vi "Test PieChart and Legend.vi"() -> ()   [LabVIEW 2020]
uses:
  Piechart Class/Pie Slice.ctl
  <vilib>/Utility/miscctls.llb/LVRowAndColumnTypeDef.ctl
  Piechart Class/PieChart.lvclass
panel:
  in  "Show/Hide Title":bool
  in  "Show/Hide Legend":bool
  in  "Selection":i32 min=-1 max=9
  out "Pie Chart":picture
  in  "Multicolumn Listbox":i32(listbox)
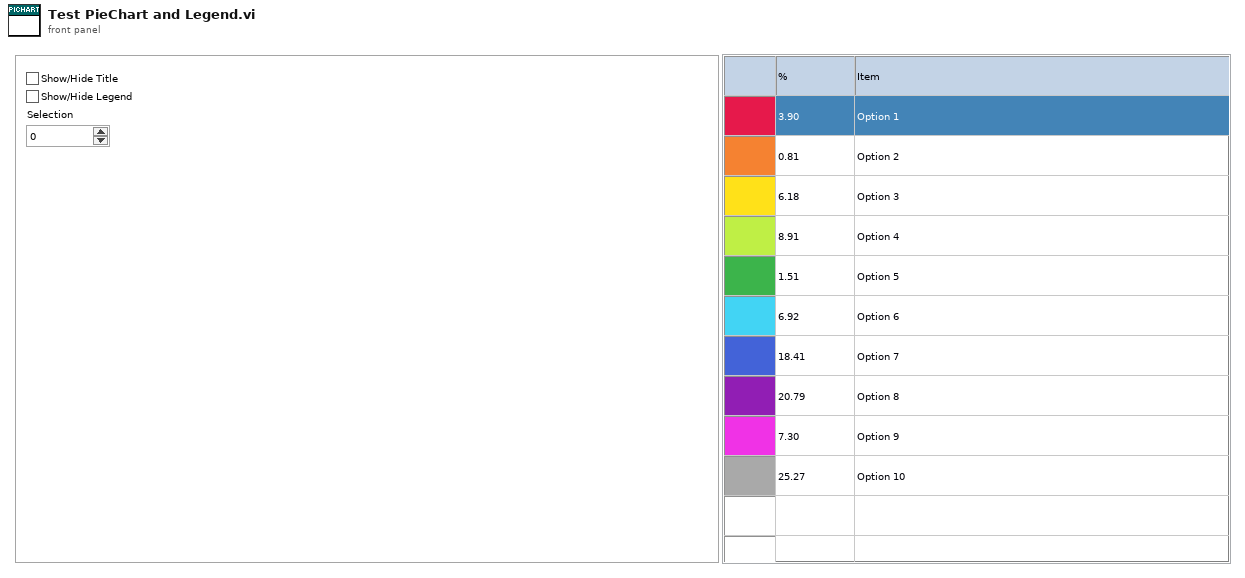
[diagram p1: front panel]
types:
  T1 = typedef "LVRowAndColumnTypeDef.ctl" = cluster{"Row":i32, "Column":i32}
  T2 = typedef "PieChart.lvclass/Pie Slice.ctl" = cluster{"Value":dbl, "Label":string}
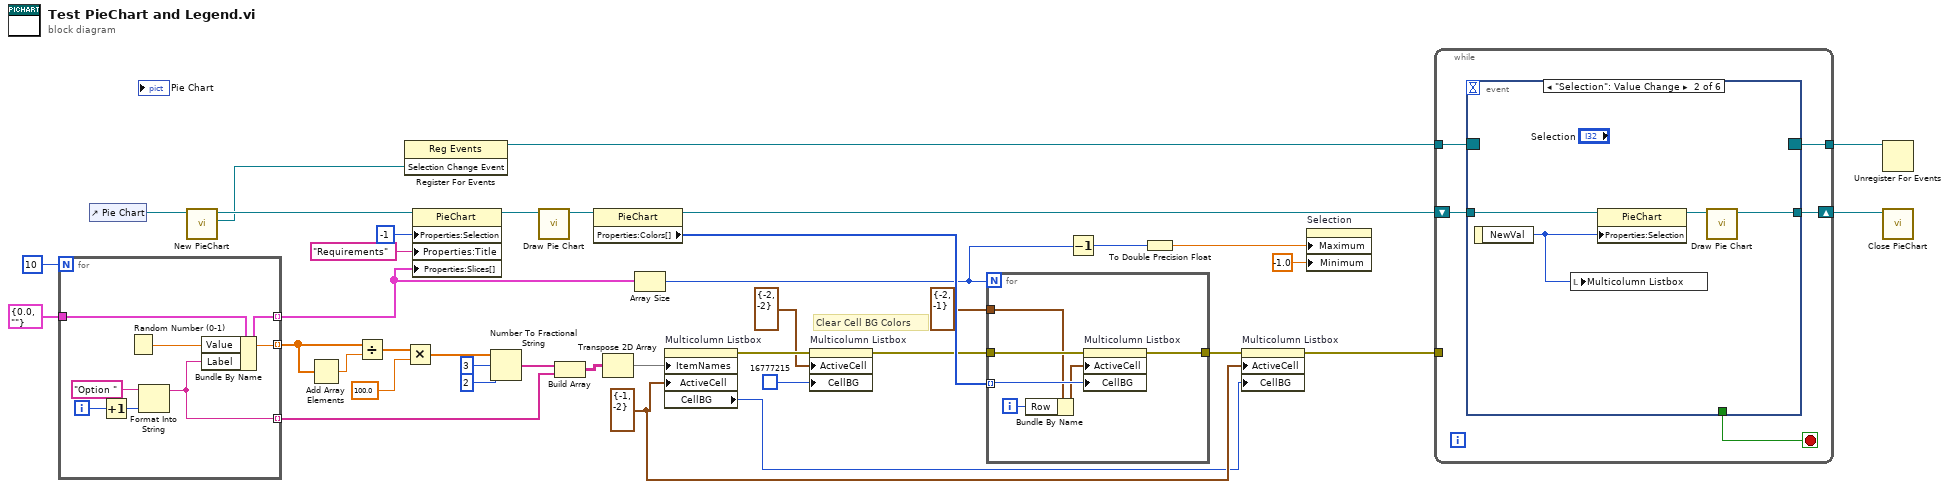
[diagram p0: block diagram]
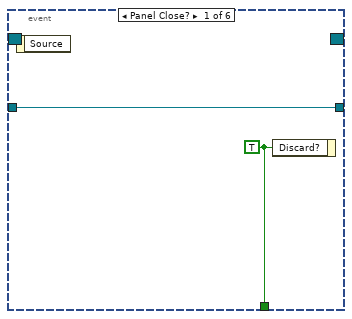
[diagram p2: hidden frame]
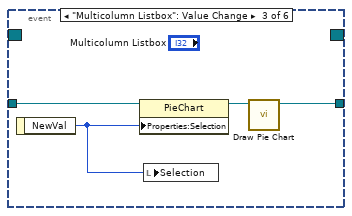
[diagram p3: hidden frame]
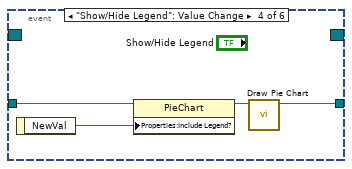
[diagram p4: hidden frame]
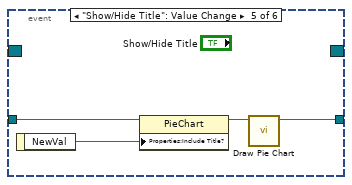
[diagram p5: hidden frame]
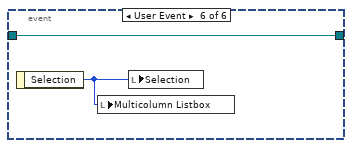
[diagram p6: hidden frame]
diagram:
  w9 = T1 {"Row"=-1, "Column"=-2} ("Active Cell:Active Cell")
  # "Clear Cell BG Colors"
  n1 = for {
    N: 10 -> [_]
    tunnel: T2 {"Value"=0.0, "Label"=""} ("Slice") -> [w46]
    tunnel: [w42] -> w6 mode=indexing
    tunnel: [w41] -> w27 mode=indexing
    tunnel: [w40] -> w18 mode=indexing
    i -> [w45]
    n2 = Increment(x=w45) -> (x+1=w44:i32)
    n3 = Random Number (0-1)() -> (number: 0 to 1=w41:dbl)
    n4 = Format Into String(initial string="Option ", w44) -> (resulting string=w40:string)  [unwired: 2 in, 1 out]
    n5 = Bundle By Name(cluster=w46, "Value"=w41, "Label"=w40) -> (w42:T2)
  }
  n6 = control-ref of="Pie Chart"() -> (w39:refnum<vi>)
  n7 = call "New PieChart.vi"("Reference"=w39) -> ("Selection Change Event"=w31:refnum<user-event>, "PieChart out"=w38:refnum<class "PieChart.lvclass">)  [unwired: 8 in, 1 out]
  n8 = Add Array Elements(numeric array=w27) -> (sum=w26:dbl)
  n9 = Divide(x=w27, y=w26) -> (x/y=w25:dbl[])
  n10 = register-events(w31) -> (reference out=w30:refnum<event-registration>)  [unwired: 2 in, 1 out]
  n11 = Multiply(x=w25, y=100.0 ("number: 0 to 1")) -> (x*y=w22:dbl[])
  n12 = property class="PieChart"(reference=w38, "Properties:Selection"=-1 ("Selection"), "Properties:Title"="Requirements" ("Title"), "Properties:Slices[]"=w6) -> (reference out=w34:refnum<class "PieChart.lvclass">)  [unwired: 1 in, 1 out]
  n13 = Number To Fractional String(number=w22, width (-)=i16 3, precision (6)=i16 2) -> (F-format string=w19:string[])  [unwired: 1 in]
  n14 = call-dynamic "Draw Pie Chart.vi"("PieChart in"=w34) -> ("PieChart out"=w33:refnum<class "PieChart.lvclass">)  [unwired: 9 in, 1 out]
  n15 = Build Array(w19, w18) -> (w17:string[][])
  n16 = property class="PieChart"(reference=w33) -> (reference out=w23:refnum<class "PieChart.lvclass">, "Properties:Colors[]"=w15:u32[])  [unwired: 1 in, 1 out]
  n17 = Transpose 2D Array(2D array=w17) -> (transposed array=w16:string[][])
  n18 = Array Size(array=w6) -> (size(s)=w4:i32)
  n19 = property on="Multicolumn Listbox" class="MCListbox (strict)"("ItemNames"=w16, "ActiveCell"=w9) -> (error out=w14:errorcluster, "CellBG"=w8:u32)  [unwired: 2 in, 1 out]
  n20 = property on="Multicolumn Listbox" class="MCListbox (strict)"(error in=w14, "ActiveCell"=T1 {"Row"=-2, "Column"=-2} ("Active Cell:Active Cell"), "CellBG"=u32 16777215) -> (error out=w13:errorcluster)  [unwired: 1 in, 1 out]
  n21 = for {
    N: w4 -> [_]
    tunnel: w13 -> [w52]
    tunnel: w15 -> [w51] mode=indexing
    tunnel: T1 {"Row"=-2, "Column"=-1} ("Active Cell:Active Cell") -> [w50]
    tunnel: [w47] -> w10
    i -> [w48]
    n22 = Bundle By Name(cluster=w50, "Row"=w48) -> (w49:T1)
    n23 = property on="Multicolumn Listbox" class="MCListbox (strict)"(error in=w52, "ActiveCell"=w49, "CellBG"=w51) -> (error out=w47:errorcluster)  [unwired: 1 in, 1 out]
  }
  n24 = Decrement(x=w4) -> (x-1=w2:i32)
  n25 = To Double Precision Float(number=w2) -> (double precision float=w3:dbl)
  n26 = property on="Multicolumn Listbox" class="MCListbox (strict)"(error in=w10, "ActiveCell"=w9, "CellBG"=w8) -> (error out=w7:errorcluster)  [unwired: 1 in, 1 out]
  n27 = property on="Selection" class="DigNum (strict)"("Maximum"=w3, "Minimum"=-1.0 ("Data Entry Limits:Minimum")) -> ()  [unwired: 2 in, 2 out]
  n28 = while {
    shift-right: [w56] -> w37
    shift-left: w23 -> [w55]
    tunnel: w30 -> [w54]
    tunnel: [w53] -> w29
    tunnel: w7 -> [_]
    stop <- w57 stop-if-true
    n29 = event shown="[1] \"Selection\": Value Change" {
      selector: w54 -> [_ _ _ _ _ _]
      dyn-events: [_ _ _ _ _ _] -> w53
      timeout: _ -> [_ _ _ _ _ _]
      tunnel: [w59 _ _ _ _ _] -> w57
      tunnel: [w58 w61 w65 w69 w73 w77] -> w56
      tunnel: w55 -> [w58 w63 w67 w71 w75 w77]
      event Panel Close? {
        w59 = TRUE ("Discard?")
        n30 = event-data() -> ()  [unwired: 1 in, 1 out]
        n31 = event-data("Discard?"=w59) -> ()  [unwired: 1 in, 1 out]
      }
      event "Selection": Value Change {
        n32 = event-data() -> ("NewVal"=w60:i32)  [unwired: 1 in]
        n33 = local write "Multicolumn Listbox"(w60) -> ()
        n34 = property class="PieChart"(reference=w63, "Properties:Selection"=w60) -> (reference out=w62:refnum<class "PieChart.lvclass">)  [unwired: 1 in, 1 out]
        n35 = call-dynamic "Draw Pie Chart.vi"("PieChart in"=w62) -> ("PieChart out"=w61:refnum<class "PieChart.lvclass">)  [unwired: 9 in, 1 out]
      }
      event "Multicolumn Listbox": Value Change {
        n36 = event-data() -> ("NewVal"=w64:i32)  [unwired: 1 in]
        n37 = property class="PieChart"(reference=w67, "Properties:Selection"=w64) -> (reference out=w66:refnum<class "PieChart.lvclass">)  [unwired: 1 in, 1 out]
        n38 = local write "Selection"(w64) -> ()
        n39 = call-dynamic "Draw Pie Chart.vi"("PieChart in"=w66) -> ("PieChart out"=w65:refnum<class "PieChart.lvclass">)  [unwired: 9 in, 1 out]
      }
      event "Show/Hide Legend": Value Change {
        n40 = event-data() -> ("NewVal"=w68:bool)  [unwired: 1 in]
        n41 = property class="PieChart"(reference=w71, "Properties:Include Legend?"=w68) -> (reference out=w70:refnum<class "PieChart.lvclass">)  [unwired: 1 in, 1 out]
        n42 = call-dynamic "Draw Pie Chart.vi"("PieChart in"=w70) -> ("PieChart out"=w69:refnum<class "PieChart.lvclass">)  [unwired: 9 in, 1 out]
      }
      event "Show/Hide Title": Value Change {
        n43 = event-data() -> ("NewVal"=w72:bool)  [unwired: 1 in]
        n44 = property class="PieChart"(reference=w75, "Properties:Include Title?"=w72) -> (reference out=w74:refnum<class "PieChart.lvclass">)  [unwired: 1 in, 1 out]
        n45 = call-dynamic "Draw Pie Chart.vi"("PieChart in"=w74) -> ("PieChart out"=w73:refnum<class "PieChart.lvclass">)  [unwired: 9 in, 1 out]
      }
      event User Event {
        n46 = event-data() -> ("Selection"=w76:i32)  [unwired: 1 in]
        n47 = local write "Multicolumn Listbox"(w76) -> ()
        n48 = local write "Selection"(w76) -> ()
      }
    }
  }
  n49 = Unregister For Events(event registration refnum=w29) -> ()  [unwired: 1 in, 1 out]
  n50 = call "Close PieChart.vi"("PieChart in"=w37) -> ()  [unwired: 10 in, 1 out]
